vi "Launch Action - TDMS Writer.vi"(8 "error in (no error)":errorcluster, 9 "CAN Configurations":T2[](array[typedef]) {"Sample Rate (Hz)" format="%#_13g"}, 10 "DAQ AI Configurations":T1[](array[typedef]) {"Terminal Config" items=["Default"=-1, "RSE"=10083, "NRSE"=10078, "Differential"=10106, "Pseudodifferential"=12529]; "Min (V)" format="%#_13g"; "Max (V)" format="%#_13g"; "Sample Rate (Hz)" format="%#_13g"}, 11 "Log file path":path) -> (0 "error out":errorcluster)   [LabVIEW 2021, in "XNET-CAN-Signal-Logger.lvlib"]
uses:
  XNET-CAN-Signal-Logger.lvlib
  Typedef/Def-CAN Port Configuration.ctl
  Typedef/Def-DAQ AI Configuration.ctl
  Global Variables.vi
  Action - TDMS Writer.vi
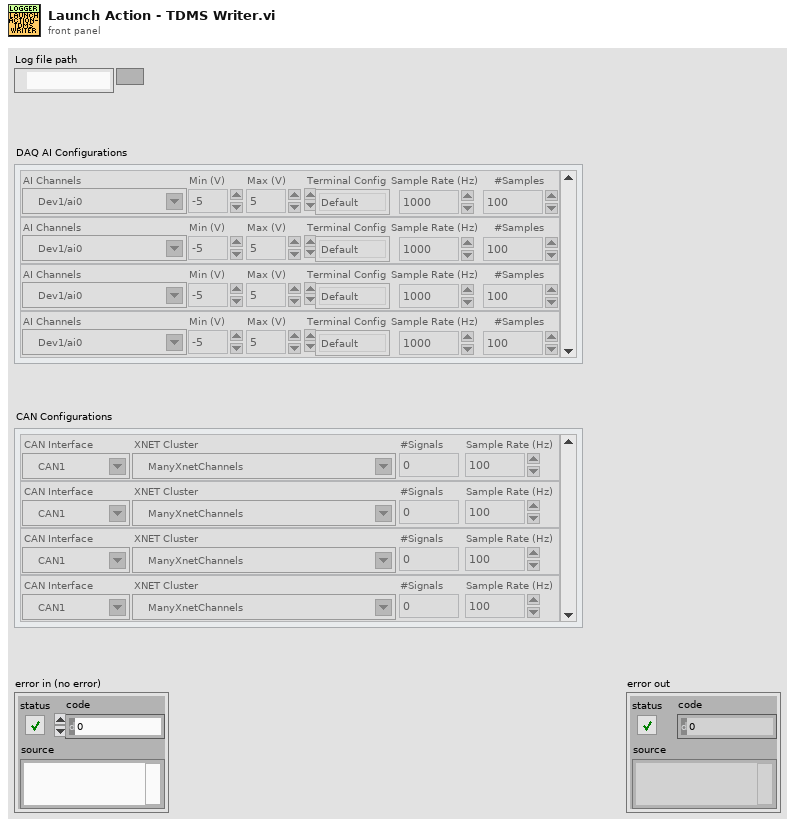
[diagram p1: front panel]
types:
  T1 = typedef "XNET-CAN-Signal-Logger.lvlib/Def-DAQ AI Configuration.ctl" = cluster{"AI Channels":tag, "Min (V)":dbl, "Max (V)":dbl, "Terminal Config":i32, "Sample Rate (Hz)":dbl, "#Samples":i32}
  T2 = typedef "XNET-CAN-Signal-Logger.lvlib/Def-CAN Port Configuration.ctl" = cluster{"CAN Interface":refnum<k21>, "XNET Cluster":refnum<k21>, "#Signals":i32, "Sample Rate (Hz)":dbl}
  T3 = enum16{"open", "open or create", "create or replace", "create", "open (read-only)"}
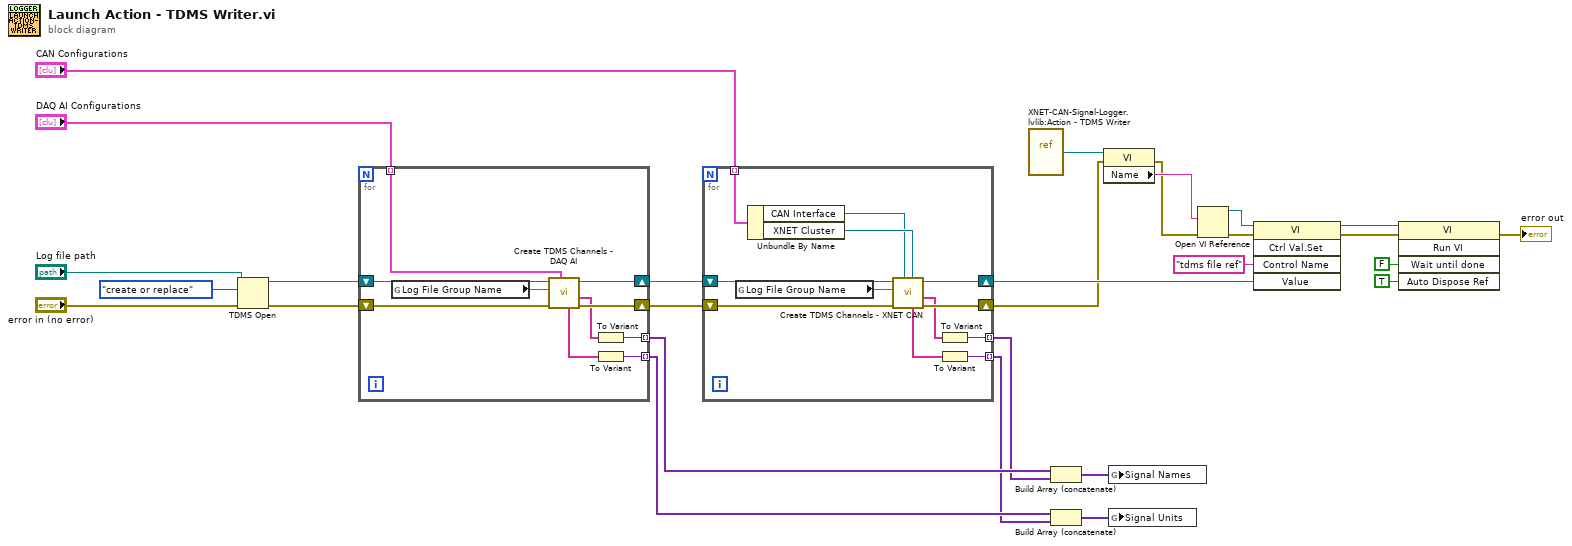
[diagram p0: block diagram]
diagram:
  n1 = TDMS Open(8:"error in (no error)", 10:T3."create or replace" ("operation (0:open)"), 11:"Log file path") -> (0:w9:errorcluster, 3:w11:refnum<k34>)  [unwired: 4 in]
  n2 = for {
    tunnel: "DAQ AI Configurations" -> [w29] mode=indexing
    shift-right: [w36] -> w10
    shift-left: w11 -> [w38]
    shift-right: [w34] -> w8
    shift-left: w9 -> [w35]
    tunnel: [w32] -> w4 mode=indexing
    tunnel: [w31] -> w3 mode=indexing
    n3 = global read "Global Variables.vi" "Log File Group Name"() -> (w37:string)
    n4 = call "Create TDMS Channels - DAQ AI.vi"("DAQ AI Configuration"=w29, "error in (no error)"=w35, "group name in"=w37, "TDMS ref in"=w38) -> ("error out"=w34:errorcluster, "Signal Names"=w30:string[], "TDMS ref out"=w36:refnum<k34>, "Signal Units"=w33:string[])  [unwired: 3 in, 1 out]
    n5 = To Variant(anything=w30) -> (Variant=w32:variant)
    n6 = To Variant(anything=w33) -> (Variant=w31:variant)
  }
  n7 = for {
    tunnel: "CAN Configurations" -> [w50] mode=indexing
    shift-right: [w45] -> w17
    shift-left: w10 -> [w47]
    shift-right: [w43] -> w15
    shift-left: w8 -> [w44]
    tunnel: [w41] -> w1 mode=indexing
    tunnel: [w40] -> w2 mode=indexing
    n8 = global read "Global Variables.vi" "Log File Group Name"() -> (w46:string)
    n9 = Unbundle By Name(w50) -> ("CAN Interface"=w48:refnum<k21>, "XNET Cluster"=w49:refnum<k21>)
    n10 = call "Create TDMS Channels - XNET CAN.vi"("XNET Cluster"=w49, "CAN Interface"=w48, "error in (no error)"=w44, "group name in"=w46, "TDMS ref in"=w47) -> ("error out"=w43:errorcluster, "Signal Names"=w39:string[], "TDMS ref out"=w45:refnum<k34>, "Signal Units"=w42:string[])  [unwired: 2 in, 1 out]
    n11 = To Variant(anything=w39) -> (Variant=w41:variant)
    n12 = To Variant(anything=w42) -> (Variant=w40:variant)
  }
  n13 = vi-ref "XNET-CAN-Signal-Logger.lvlib:Action - TDMS Writer.vi"() -> (w28:refnum<vi>)
  n14 = Build Array (concatenate)(w4, w1) -> (w6:variant[])
  n15 = Build Array (concatenate)(w3, w2) -> (w5:variant[])
  n16 = property class="VI"(reference=w28, error in=w15) -> (error out=w26:errorcluster, "Name"=w27:string)  [unwired: 1 out]
  n17 = global write "Global Variables.vi" "Signal Names"(w6) -> ()
  n18 = global write "Global Variables.vi" "Signal Units"(w5) -> ()
  n19 = Open VI Reference(vi path=w27, error in (no error)=w26) -> (vi reference=w20:refnum<vi>, error out=w22:errorcluster)  [unwired: 4 in]
  n20 = invoke class="VI" method="Ctrl Val.Set"(reference=w20, error in=w22, "Control Name"="tdms file ref", "Value"=w17) -> (reference out=w14:refnum<vi>, error out=w13:errorcluster)  [unwired: 1 in, 3 out]
  n21 = invoke class="VI" method="Run VI"(reference=w14, error in=w13, "Wait until done"=FALSE ("Wait Until Done"), "Auto Dispose Ref"=TRUE ("Auto Dispose Reference")) -> (error out=→"error out":errorcluster)  [unwired: 1 in, 4 out]
